vi "Implement IIR Direct Filter.vi"   [LabVIEW 2020, in "NI_MAPro.lvlib"]
uses:
  NI_MAPro.lvlib
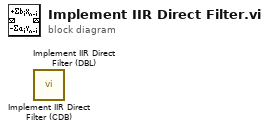
[diagram p0: block diagram]
diagram:
  n1 = call "Implement IIR Direct Filter (CDB).vi"() -> ()  [unwired: 5 in, 2 out]
  n2 = call "Implement IIR Direct Filter (DBL).vi"() -> ()  [unwired: 5 in, 2 out]
